vi "Acquire PDM Waveform.vi"(11 "ObjRefIn":u32) -> (0 "error out":errorcluster, 1 "Y":dbl[](array[numeric]), 3 "dt":dbl)   [LabVIEW 2021]
uses:
  <vilib>/PDM Acquisition Toolkit/host/Classes/Tasks/PCM Input/Controls/DVR PCM Input Task.ctl
  <vilib>/PDM Acquisition Toolkit/host/Classes/Tasks/PCM Input/PCM Input Task.lvclass
  <vilib>/PDM Acquisition Toolkit/host/API/Public/Start/Start PCM Input Task.vi
  <vilib>/PDM Acquisition Toolkit/host/API/Public/Read/Read PCM Input Waveform.vi
  <vilib>/PDM Acquisition Toolkit/host/API/Public/Stop/Stop PCM Input Task.vi
  <vilib>/PDM Acquisition Toolkit/host/API/Public/Clear/Clear PCM Input Task.vi
  <vilib>/PDM Acquisition Toolkit/host/API/PDM Acquisition Toolkit.lvlib
panel:
  out "Waveform Graph":waveform(dbl)(graph)
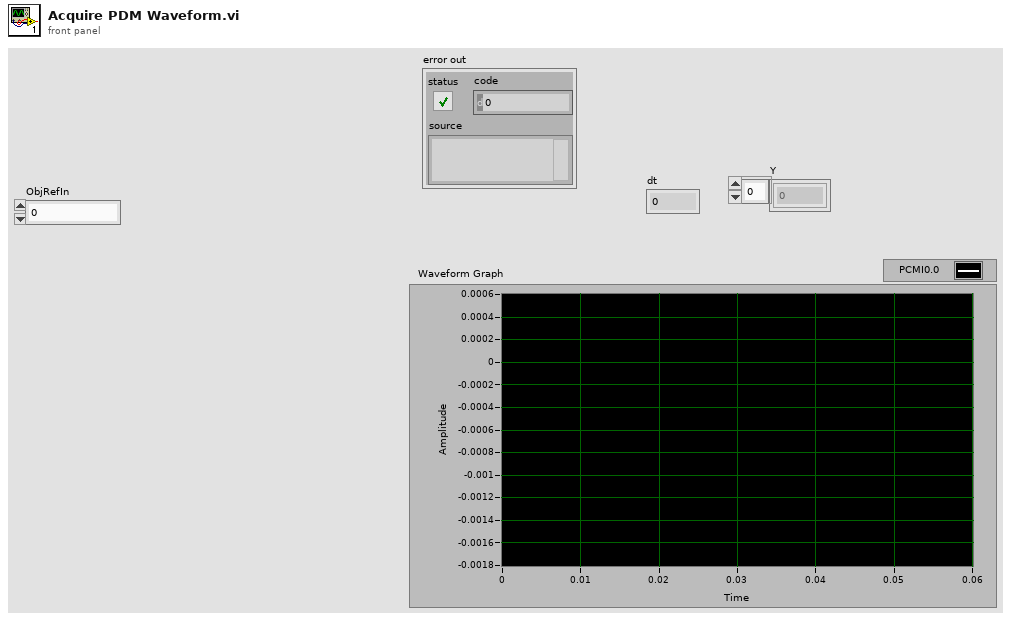
[diagram p1: front panel]
types:
  T1 = typedef "PDM Acquisition Class Library.lvlib/PCM Input Task.lvclass/DVR PCM Input Task.ctl" = refnum<data-value>
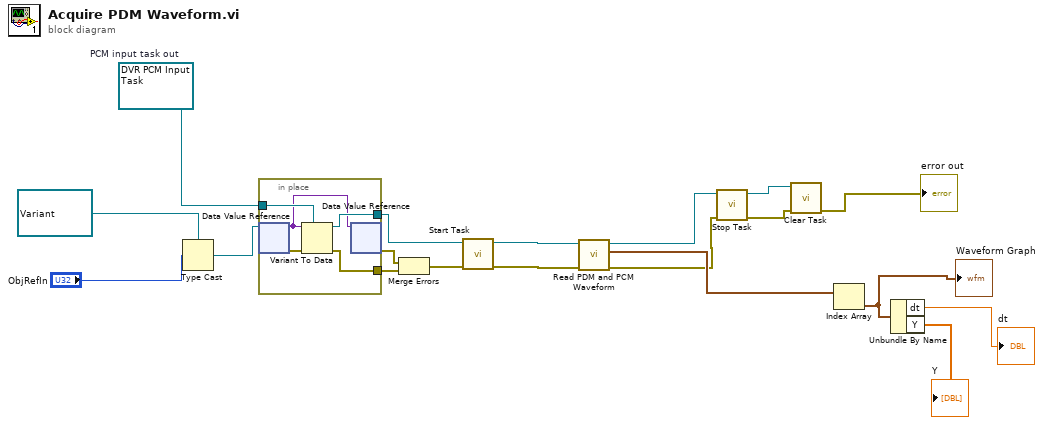
[diagram p0: block diagram]
diagram:
  w14 = T1 refnum  # PCM input task out
  n1 = Type Cast(type=refnum<data-value> refnum ("data value reference"), x="ObjRefIn") -> (*(type *) &x=w12:refnum<data-value>)
  n2 = in-place {
    in-place-border: [w24] -> w13
    in-place-border: [w22] -> w17
    in-place-border: w14 -> [w21]
    n3 = in-place-dvr #1(w12) -> (w20:variant, w23:errorcluster)
    n4 = Variant To Data(error in=w23, type=w21, Variant=w20) -> (data=w24:T1, error out=w22:errorcluster)
    n5 = in-place-dvr #1(w20) -> (w18:errorcluster)  [unwired: 1 out]
  }
  n6 = Merge Errors(w18, w17) -> (w16:errorcluster)
  n7 = call-poly <vilib>:"Start Task.vi"("error in"=w16, "PCM input task in"=w13) -> ("error out"=w19:errorcluster, "PCM input task out"=w15:T1)  [unwired: 8 in]
  n8 = call-poly <vilib>:"Read PDM and PCM Waveform.vi"("error in"=w19, "PCM input task In"=w15) -> ("error out"=w3:errorcluster, "PCM waveforms"=w10:waveform(dbl)[], "PCM input task out"=w5:T1)  [unwired: 4 in, 3 out]
  n9 = call-poly <vilib>:"Stop Task.vi"("error in"=w3, "PCM input task In"=w5) -> ("error out"=w2:errorcluster, "PCM input task out"=w4:T1)  [unwired: 8 in]
  n10 = call-poly <vilib>:"Clear Task.vi"("error in"=w2, "PCM input task in"=w4) -> ("error out"=→"error out":errorcluster)  [unwired: 9 in]
  n11 = Index Array(array=w10) -> (element=w8:waveform(dbl))  [unwired: 1 in]
  "Waveform Graph" <- w8
  n12 = Unbundle By Name(w8) -> ("dt"=→"dt":dbl, "Y"=→"Y":dbl[])
